vi "Test SplashWindow2.vi"   [LabVIEW 2020]
uses:
  a3eb0aa5-2cc5-4148-8f17-44e3bf90e6b5.vi
  a3eb0aa5-2cc5-4148-8f17-44e3bf90e6b5.vi/1b47866c-8e2d-43a7-815f-8cf18635e5a1.vi
  <userlib>/_NEVSTOP/TagDB/_Support/Change Detector/TagDB dbChanged.vi
  <userlib>/_NEVSTOP/TagDB/_Support/Error/_Clear Errors.vi
  a3eb0aa5-2cc5-4148-8f17-44e3bf90e6b5.vi/1b47866c-8e2d-43a7-815f-8cf18635e5a1.vi/29b2ea6d-6d7f-4e4a-ad31-a5cb760462c7.vi
  <userlib>/_NEVSTOP/TagDB/API/TagDB-Status.vi
  <userlib>/_NEVSTOP/TagDB/_Support/Change Detector/TagDB ChangeFlag.vi
  <userlib>/_NEVSTOP/TagDB/_Support/DataAccess/_NameCacher.vi
  <userlib>/_NEVSTOP/TagDB/_Support/Error/_[error50002]Invalid DataType.vi
  <userlib>/_NEVSTOP/TagDB/_Support/Error/_[error50000]Invalid DB REF.vi
  <userlib>/_NEVSTOP/TagDB/_Support/DataAccess/TagDB Ref to DVR.vi
  <userlib>/_NEVSTOP/TagDB/_Support/URL/TRIM-BOTH-SPACE.vi
  <userlib>/_NEVSTOP/TagDB/_Support/Error/_Build Error Cluster.vi
  <userlib>/_NEVSTOP/Communicable State Machine(CSM)/Communicable State Machine.lvlib
  <userlib>/_NEVSTOP/TagDB/Add-ons/RefManager/TagDB RefManager.lvlib
  <userlib>/_NEVSTOP/TagDB/TagDB.lvlib
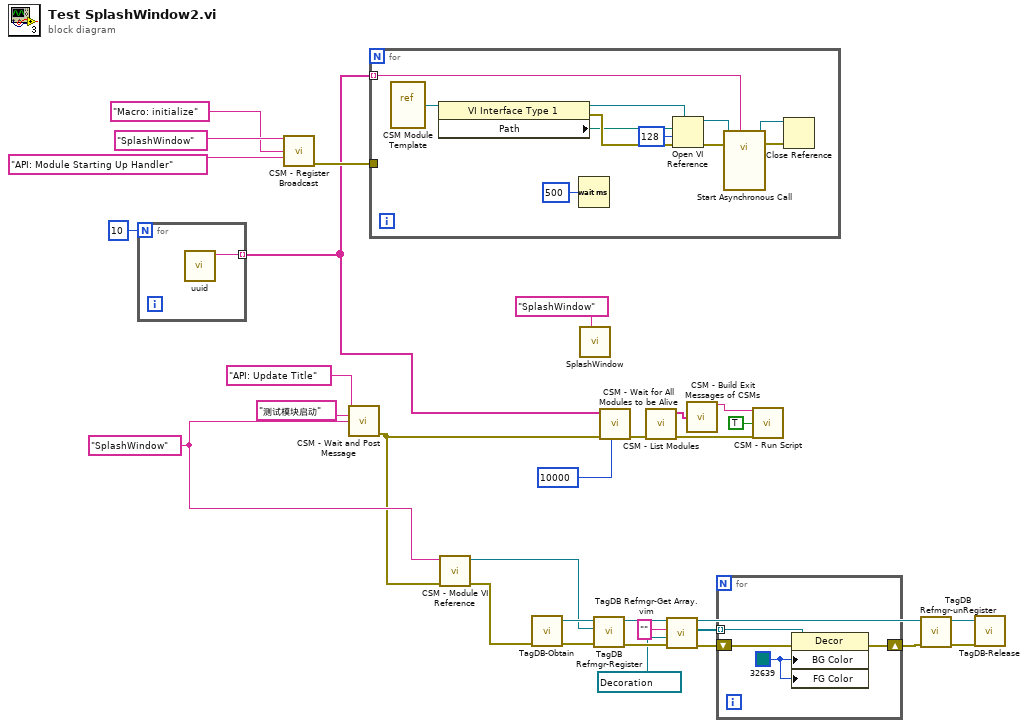
[diagram p0: block diagram]
diagram:
  w14 = "SplashWindow" ("Name (\"\" to Use UUID)")
  n1 = for {
    N: 10 -> [_]
    tunnel: [w32] -> w2 mode=indexing
    n2 = call <userlib>:"uuid.vi"() -> ("UUID"=w32:string)  [unwired: 11 in]
  }
  n3 = call <userlib>:"CSM - Register Broadcast.vi"("CSM Name(Empty for Broadcast Event)"="SplashWindow" ("Name (\"\" to Use UUID)"), "Trigger"="Macro: initialize" ("Name (\"\" to Use UUID)"), "API (If \"\", Same as Trigger)"="API: Module Starting Up Handler" ("API (If \"\", Same as Trigger)")) -> ("error out"=w13:errorcluster)  [unwired: 11 in, 1 out]
  n4 = call <userlib>:"CSM - Wait and Post Message.vi"("State"="API: Update Title", "Arguments (\"\")"="测试模块启动" ("State"), "Target Module"=w14) -> ("error out"=w4:errorcluster)  [unwired: 11 in, 1 out]
  n5 = for {
    tunnel: w13 -> [_]
    tunnel: w2 -> [w33] mode=indexing
    n6 = vi-ref <userlib>:"CSM Module Template.vi"() -> (w36:refnum<vi>)
    n7 = property class="VI Interface Type 1"(reference=w36) -> (reference out=w40:refnum<vi>, error out=w38:errorcluster, "Path"=w37:path)  [unwired: 1 in]
    n8 = Wait (ms)(milliseconds to wait=u32 500) -> ()  [unwired: 1 out]
    n9 = Open VI Reference(type specifier VI Refnum (for type only)=w40, vi path=w37, options=128, error in (no error)=w38) -> (vi reference=w39:refnum<vi>, error out=w35:errorcluster)  [unwired: 2 in]
    n10 = call-by-ref "Start Asynchronous Call"(reference=w39, error in=w35, "Name (\"\" to Use UUID)"=w33) -> (reference out=w42:refnum<vi>, error out=w41:errorcluster)  [unwired: 11 in]
    n11 = Close Reference(reference=w42, error in (no error)=w41) -> ()  [unwired: 1 out]
  }
  n12 = call <userlib>:"CSM - Module VI Reference.vi"("error in (no error)"=w4, "CSM Name"=w14) -> ("error out"=w15:errorcluster, "CSM Module VIRef"=w27:refnum<vi>)  [unwired: 8 in]
  n13 = call <userlib>:"TagDB-Obtain.vi"("error in (no error)"=w15) -> ("error out"=w26:errorcluster, "TagDB"=w28:refnum<k1>)  [unwired: 4 in, 1 out]
  n14 = call "SplashWindow.vi"("Name (\"\" to Use UUID)"="SplashWindow" ("Name (\"\" to Use UUID)")) -> ()  [unwired: 11 in]
  n15 = call <userlib>:"TagDB Refmgr-Register.vi"("error in (no error)"=w26, "VI Refnum"=w27, "TagDB in"=w28) -> ("error out"=w24:errorcluster, "TagDB out"=w25:refnum<k1>)  [unwired: 6 in, 1 out]
  n16 = call <userlib>:"CSM - Wait for All Modules to be Alive.vi"("Wait (5000 ms)"=u32 10000, "Error In"=w4, "CSM Names"=w2) -> ("error out"=w3:errorcluster)  [unwired: 6 in, 2 out]
  n17 = call <userlib>:"CSM - List Modules.vi"("Error In"=w3) -> ("error out"=w6:errorcluster, "Module Names"=w9:string[])  [unwired: 9 in]
  n18 = call "TagDB Refmgr-Get Array.vim"("error in (no error)"=w24, "Type"=refnum<vi> refnum, "RegExp"="", "DB Ref"=w25) -> ("error out"=w19:errorcluster, "References"=w17:refnum<vi>[], "DB Ref(dup)"=w18:refnum<k1>)  [unwired: 4 in, 1 out]
  n19 = call <userlib>:"CSM - Build Exit Messages of CSMs.vi"("CSMs"=w9) -> ("States"=w8:string)  [unwired: 14 in]
  n20 = for {
    shift-right: [w46] -> w20
    shift-left: w19 -> [w47]
    tunnel: w17 -> [w45] mode=indexing
    w44 = u32 32639 ("Colors:BG Color")
    n21 = property class="Decor"(reference=w45, error in=w47, "BG Color"=w44, "FG Color"=w44) -> (error out=w46:errorcluster)  [unwired: 1 out]
  }
  n22 = call <userlib>:"CSM - Run Script.vi"("CSM Scripts"=w8, "Continue If Error? (F)"=TRUE, "error in (no error)"=w6) -> ()  [unwired: 10 in, 3 out]
  n23 = call <userlib>:"TagDB Refmgr-unRegister.vi"("error in (no error)"=w20, "TagDB in"=w18) -> ("error out"=w22:errorcluster, "TagDB out"=w21:refnum<k1>)  [unwired: 8 in]
  n24 = call <userlib>:"TagDB-Release.vi"("error in (no error)"=w22, "TagDB"=w21) -> ()  [unwired: 9 in, 1 out]
